vi "FLL_PID.vi"(8 "error in (no error)":errorcluster, 11 "DSP.lvclass":refnum<class "DSP.lvclass">) -> (0 "error out":errorcluster, 2 "frequency output (Hz)":dbl, 3 "DSP.lvclass":refnum<class "DSP.lvclass">)   [LabVIEW 2019, in "DSP.lvclass"]
doc: "Please ensure that at least one period is generated or else the measurement VIs do not work properly."
uses:
  DSP.lvclass
  DSP.lvclass/DSP.ctl
  <vilib>/Waveform/WDTOps.llb/WDT Number of Waveform Samples DBL.vi
  <vilib>/PRIrvin/XY Utilities/subVIs/Circular Buffer (waveform).vi
  <vilib>/measure/matone.llb/Extract Single Tone Information 1 Chan.vi
  <vilib>/addons/control/pid/pid.llb/PID (DBL).vi
  <vilib>/addons/control/pid/NI_PID_pid.lvlib
  <vilib>/measure/NI_MAPro.lvlib
  <vilib>/PRIrvin/XY Utilities/xy_utilities.lvlib
panel:
  out "Error Chart":dbl(graph)
  in  "PID gains (Frequency)":T1={"proportional gain (Kc)"=0.3, "integral time (Ti, min)"=0.002, "derivative time (Td, min)"=0.0} {"derivative time (Td, min)" format="%.3f"; "integral time (Ti, min)" format="%.3f"; "proportional gain (Kc)" format="%.3f"}
  out "Frequency Chart":cluster{"detected frequency":dbl, dbl}(graph)
  out "process frequency":dbl format="%.2p"
  out "set point frequency":dbl format="%.2p"
  out "Waveform Graph":waveform(dbl)[](graph)
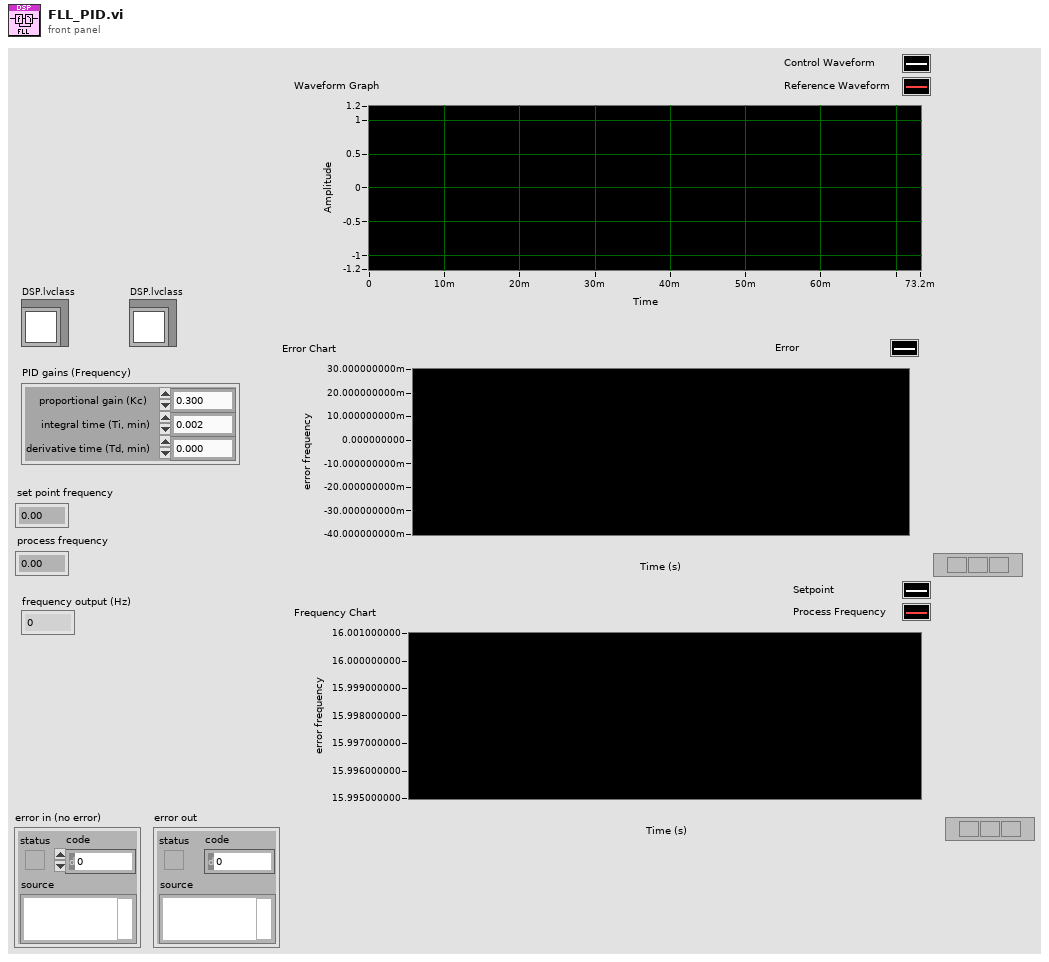
[diagram p1: front panel]
types:
  T1 = cluster{"proportional gain (Kc)":dbl, "integral time (Ti, min)":dbl, "derivative time (Td, min)":dbl}
  T2 = typedef "DSP.lvclass/REF.Channel--Cluster--Array.ctl" = T3[]
  T3 = typedef "DSP.lvclass/REF.Channel--Cluster.ctl" = cluster{"Enable?":bool, "Channel":i32, "Frequency":dbl, "Phase":dbl, "TC":dbl, "Roll-Off":i32}
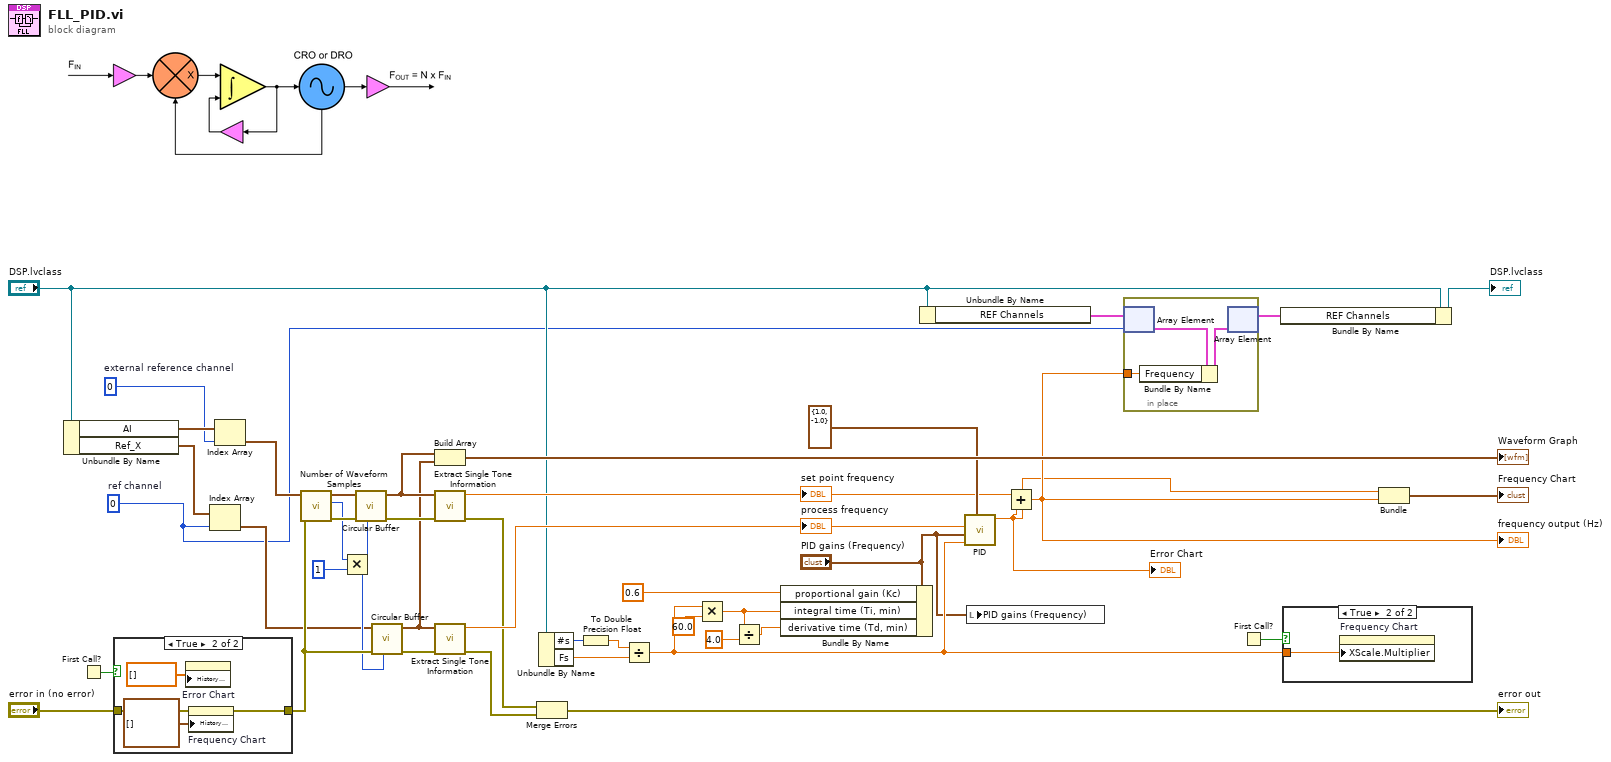
[diagram p0: block diagram]
diagram:
  w2 = 0  # external reference channel
  w1 = 0  # ref channel
  n1 = Unbundle By Name("DSP.lvclass") -> ("AI"=w6:waveform(dbl)[], "Ref_X"=w4:waveform(dbl)[])
  n2 = First Call?() -> (First Call?: T/F=w39:bool)
  n3 = case shown="True" w39 {
    tunnel: "error in (no error)" -> [w44 w48]
    tunnel: [w44 w47] -> w14
    frame False {
    }
    frame True {
      n4 = property on="Error Chart" class="WFChart (strict)"("History Data"=dbl[] []) -> ()  [unwired: 2 in, 2 out]
      n5 = property on="Frequency Chart" class="WFChart (strict)"(error in=w48, "History Data"=cluster{"detected frequency":dbl, dbl}[] []) -> (error out=w47:errorcluster)  [unwired: 1 in, 1 out]
    }
  }
  n6 = Index Array(array=w4, index=w1) -> (element=w3:waveform(dbl))
  n7 = Index Array(array=w6, index=w2) -> (element=w5:waveform(dbl))
  n8 = call-poly <vilib>:"Number of Waveform Samples.vi"("error in (no error)"=w14, "waveform in"=w5) -> ("error out"=w16:errorcluster, "number of samples"=w8:i32, "waveform out"=w15:waveform(dbl))  [unwired: 7 in]
  n9 = Multiply(x=w8, y=1) -> (x*y=w12:i32)
  n10 = call-poly <vilib>:"Circular Buffer.vi"("History Length [1024]"=w12, "error in"=w16, "Waveform in"=w15) -> ("error out"=w17:errorcluster, "Waveform out"=w11:waveform(dbl))  [unwired: 7 in]
  n11 = call-poly <vilib>:"Circular Buffer.vi"("History Length [1024]"=w12, "error in"=w14, "Waveform in"=w3) -> ("error out"=w18:errorcluster, "Waveform out"=w10:waveform(dbl))  [unwired: 7 in]
  n12 = Build Array(w11, w10) -> (→"Waveform Graph":waveform(dbl)[])
  n13 = call-poly <vilib>:"Extract Single Tone Information.vi"("error in (no error)"=w17, "time signal in"=w11) -> ("error out"=w19:errorcluster, "detected frequency"=w9:dbl)  [unwired: 4 in, 4 out]
  "set point frequency" <- w9
  n14 = call-poly <vilib>:"Extract Single Tone Information.vi"("error in (no error)"=w18, "time signal in"=w10) -> ("error out"=w42:errorcluster, "detected frequency"=w33:dbl)  [unwired: 4 in, 4 out]
  "process frequency" <- w33
  n15 = Merge Errors(w19, w42) -> (→"error out":errorcluster)
  n16 = Unbundle By Name("DSP.lvclass") -> ("#s"=w35:i32, "Fs"=w34:dbl)
  n17 = To Double Precision Float(number=w35) -> (double precision float=w36:dbl)
  n18 = Divide(x=w36, y=w34) -> (x/y=w29:dbl)
  n19 = Multiply(x=w29, y=60.0 ("proportional gain (Kc)")) -> (x*y=w27:dbl)
  n20 = Divide(x=w27, y=4.0) -> (x/y=w25:dbl)
  n21 = Bundle By Name(cluster="PID gains (Frequency)", "proportional gain (Kc)"=0.6, "integral time (Ti, min)"=w27, "derivative time (Td, min)"=w25) -> ()  [unwired: 1 out]
  n22 = Unbundle By Name("DSP.lvclass") -> ("REF Channels"=w22:T2)
  n23 = call-poly <vilib>:"PID.vi"("output range"=cluster{"output high":dbl, "output low":dbl} {"output high"=1.0, "output low"=-1.0}, "dt (s)"=w29, "PID gains"="PID gains (Frequency)", "process variable"=w33, "setpoint"=w9) -> ("output"=w23:dbl)  [unwired: 5 in, 1 out]
  "Error Chart" <- w23
  n24 = local write "PID gains (Frequency)"("PID gains (Frequency)") -> ()
  n25 = Add(x=w9, y=w23) -> (x+y=w20:dbl)
  "frequency output (Hz)" <- w20
  n26 = in-place {
    in-place-border: w20 -> [w49]
    n27 = in-place-array #1(w22, w1) -> (w50:T3)
    n28 = Bundle By Name(cluster=w50, "Frequency"=w49) -> (w51:T3)
    n29 = in-place-array #1(w51) -> (w21:T2)  [unwired: 1 out]
  }
  n30 = First Call?() -> (First Call?: T/F=w31:bool)
  n31 = Bundle By Name(cluster="DSP.lvclass", "REF Channels"=w21) -> (→"DSP.lvclass":refnum<class "DSP.lvclass">)
  n32 = case shown="True" w31 {
    tunnel: w29 -> [_ w52]
    frame False {
    }
    frame True {
      n33 = property on="Frequency Chart" class="WFChart (strict)"("XScale.Multiplier"=w52) -> ()  [unwired: 2 in, 2 out]
    }
  }
  n34 = Bundle("detected frequency"=w9, w20) -> (→"Frequency Chart":cluster{"detected frequency":dbl, dbl})  [unwired: 1 in]
